vi "Print Debug Line.vi"(6 "Append newline? (T)":bool=TRUE, 7 "Add to log file? (F)":bool, 8 "error in":errorcluster, 10 "Message":string, 11 "Custom Device API in":refnum<class "Custom Device API.lvclass">) -> (0 "error out":errorcluster, 3 "Custom Device API out":refnum<class "Custom Device API.lvclass">)   [LabVIEW 2027, in "Custom Device Interfaces.lvlib" / "Custom Device API.lvclass"]
uses:
  Custom Device API.lvclass
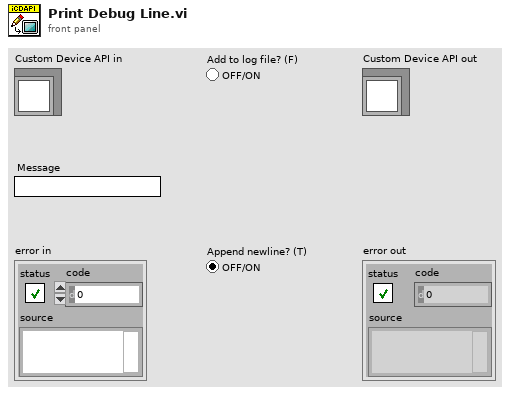
[diagram p1: front panel]
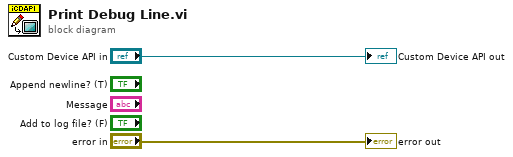
[diagram p0: block diagram]
diagram:
  "error out" <- "error in"
  "Custom Device API out" <- "Custom Device API in"
